vi "CRYCursor move in Cursor Table.vi"(8 "NewVal":string[][](array[string]), 9 "OldVal":string[][](array[string]), 10 "Cursor Coords":T1, 11 "pGraph VI":refnum<vi>) -> (3 "NewVal Out":string[][](array[string]))   [LabVIEW 2013]
uses:
  <vilib>/Utility/miscctls.llb/LVPoint32TypeDef.ctl
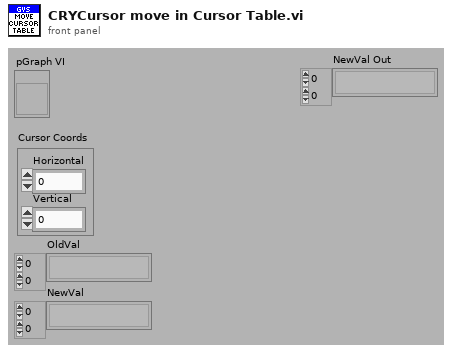
[diagram p1: front panel]
types:
  T1 = typedef "LVPoint32TypeDef.ctl" = cluster{"Horizontal":i32, "Vertical":i32}
  T2 = typedef "LVRowAndColumnTypeDef.ctl" = cluster{"Row":i32, "Column":i32}
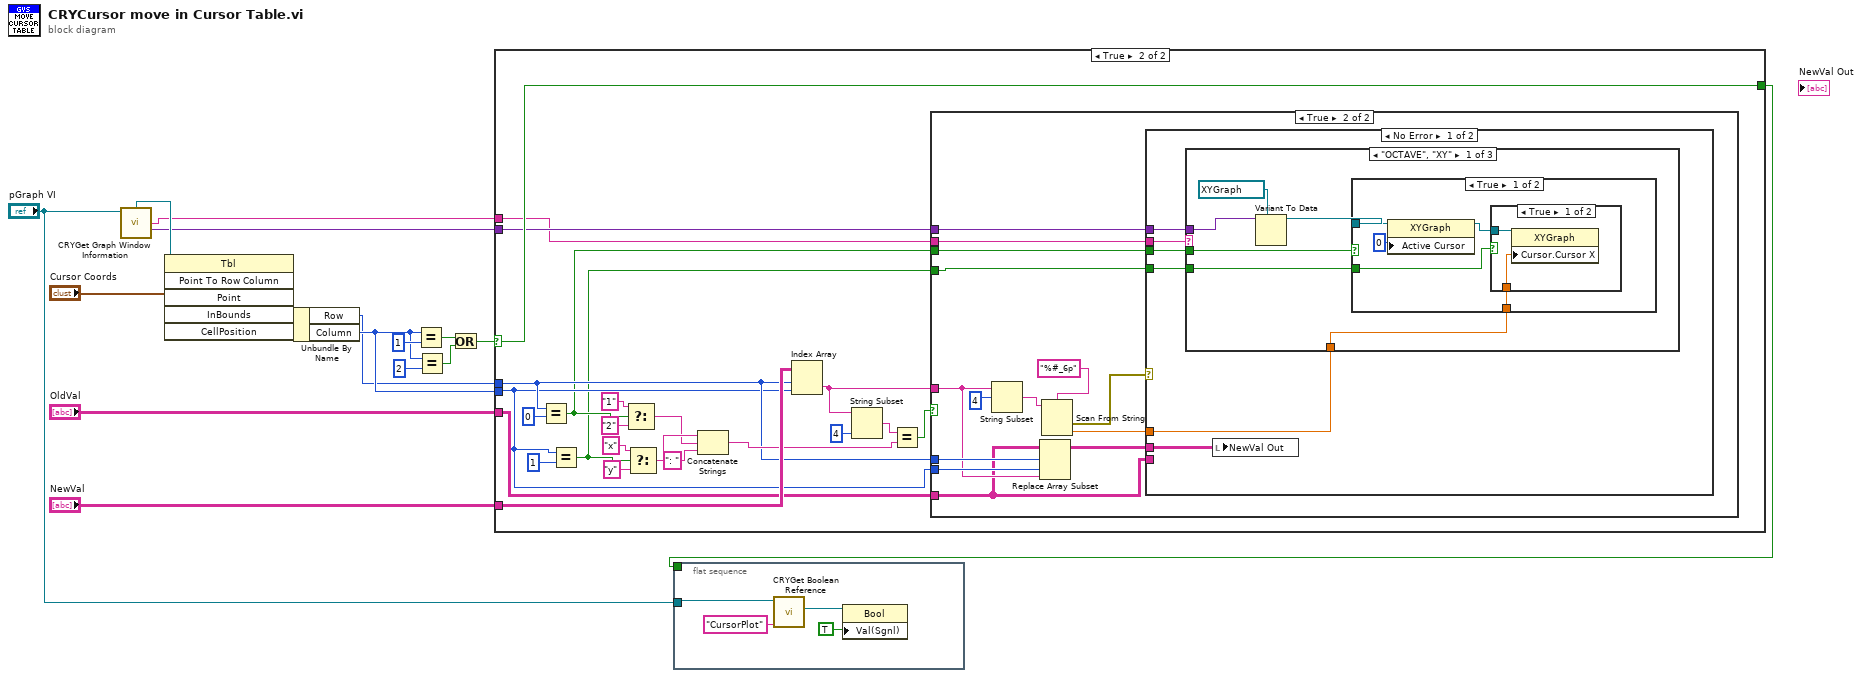
[diagram p0: block diagram]
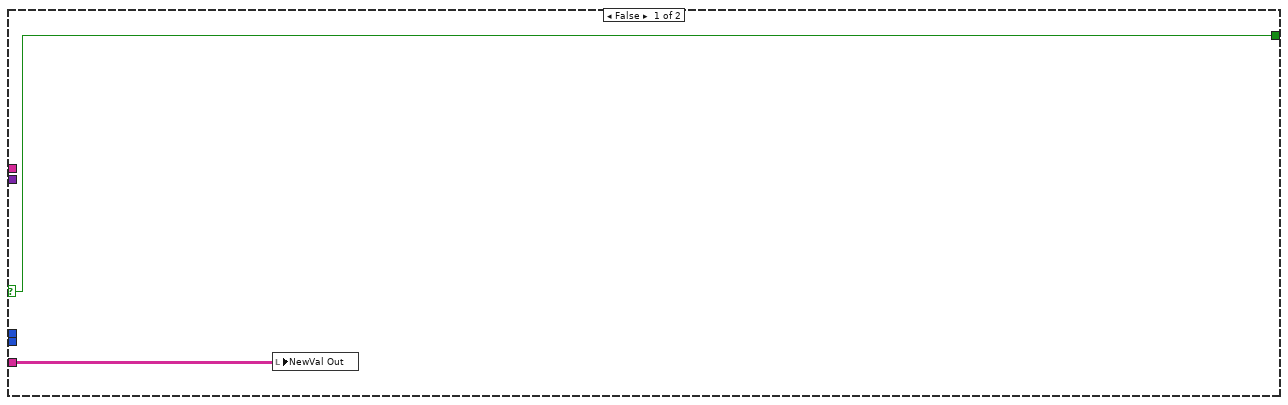
[diagram p2: hidden frame]
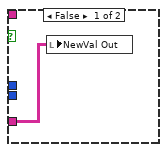
[diagram p3: hidden frame]
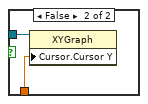
[diagram p4: hidden frame]
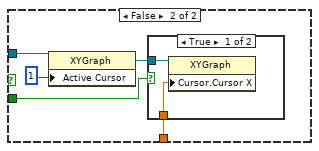
[diagram p5: hidden frame]
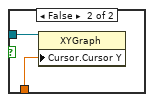
[diagram p6: hidden frame]
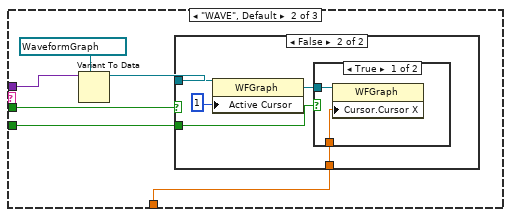
[diagram p7: hidden frame]
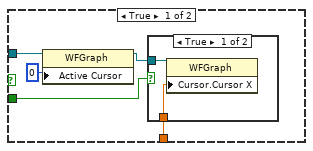
[diagram p8: hidden frame]
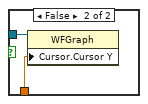
[diagram p9: hidden frame]
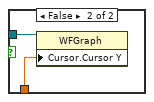
[diagram p10: hidden frame]
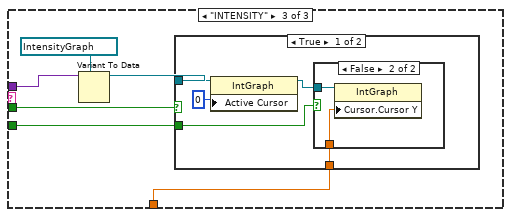
[diagram p11: hidden frame]
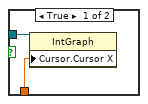
[diagram p12: hidden frame]
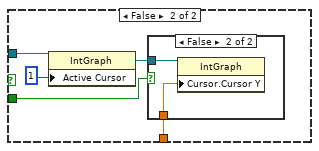
[diagram p13: hidden frame]
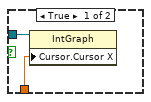
[diagram p14: hidden frame]
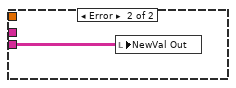
[diagram p15: hidden frame]
diagram:
  n1 = call "CRYGet Graph Window Information.vi"("pGraph VI In"="pGraph VI") -> ("Cursor Ref Out"=w5:refnum<vi>, "Graph Type Out"=w1:string, "Graph Control Ref Out"=w4:variant)  [unwired: 4 in, 8 out]
  n2 = invoke class="Tbl" method="Point To Row Column"(reference=w5, "Point"="Cursor Coords") -> ("CellPosition"=w11:T2)  [unwired: 4 in, 5 out]
  n3 = Unbundle By Name(w11) -> ("Row"=w12:i32, "Column"=w13:i32)
  n4 = Equal?(x=w13, y=1) -> (x = y?=w10:bool)
  n5 = Equal?(x=w13, y=2) -> (x = y?=w9:bool)
  n6 = Or(x=w10, y=w9) -> (x .or. y?=w16:bool)
  n7 = case shown="True" w16 {
    selector: w16 -> [w17 w24]
    tunnel: "NewVal" -> [_ w41]
    tunnel: w12 -> [_ w27]
    tunnel: w13 -> [_ w26]
    tunnel: "OldVal" -> [w18 w25]
    tunnel: [w17 w24] -> w2
    tunnel: w4 -> [_ w20]
    tunnel: w1 -> [_ w19]
    frame False {
      n8 = local write "NewVal Out"(w18) -> ()
    }
    frame True {
      n9 = Equal?(x=w27, y=0) -> (x = y?=w22:bool)
      n10 = Equal?(x=w26, y=1) -> (x = y?=w21:bool)
      n11 = Select(t="1", s=w22, f="2") -> (s? t:f=w33:string)
      n12 = Select(t="x", s=w21, f="y") -> (s? t:f=w34:string)
      n13 = Concatenate Strings(w34, w33, ": " ("string")) -> (w29:string)
      n14 = Index Array(array=w41, index (row)=w27, index (col)=w26) -> (element=w31:string)
      n15 = String Subset(string=w31, length (rest)=4 ("length (rest)")) -> (substring=w23:string)  [unwired: 1 in]
      n16 = Equal?(x=w23, y=w29) -> (x = y?=w28:bool)
      n17 = case shown="True" w28 {
        tunnel: w31 -> [_ w53]
        tunnel: w27 -> [_ w55]
        tunnel: w26 -> [_ w54]
        tunnel: w25 -> [w42 w43]
        tunnel: w22 -> [_ w49]
        tunnel: w21 -> [_ w48]
        tunnel: w19 -> [_ w46]
        tunnel: w20 -> [_ w45]
        frame False {
          n18 = local write "NewVal Out"(w42) -> ()
        }
        frame True {
          n19 = String Subset(string=w53, offset (0)=4) -> (substring=w51:string)  [unwired: 1 in]
          n20 = Replace Array Subset(array=w43, new element=w53, index (row)=w55, index (col)=w54) -> (w56:string[][])
          n21 = Scan From String(format string="%#_6p", input string=w51) -> (error out=w44:errorcluster, output 1=w47:dbl)  [unwired: 3 in, 2 out]
          n22 = case shown="No Error" w44 {
            tunnel: w56 -> [w62 _]
            tunnel: w49 -> [w61 _]
            tunnel: w48 -> [w60 _]
            tunnel: w47 -> [w59 _]
            tunnel: w46 -> [w58 _]
            tunnel: w45 -> [w57 _]
            tunnel: w43 -> [_ w135]
            frame No Error {
              n23 = case shown="\"OCTAVE\", \"XY\"" w58 {
                tunnel: w61 -> [w68 w92 w116]
                tunnel: w60 -> [w67 w91 w115]
                tunnel: w59 -> [w66 w90 w114]
                tunnel: w57 -> [w64 w88 w112]
                frame "OCTAVE", "XY" {
                  n24 = Variant To Data(type=refnum<vi> refnum ("GMListbox"), Variant=w64) -> (data=w63:refnum<vi>)  [unwired: 1 in, 1 out]
                  n25 = case shown="True" w68 {
                    tunnel: w67 -> [w71 w80]
                    tunnel: w66 -> [w73 w82]
                    tunnel: w63 -> [w70 w79]
                    frame True {
                      n26 = property on="Property Node" class="XYGraph"(reference=w70, "Active Cursor"=u32 0) -> (reference out=w69:refnum<vi>)  [unwired: 1 in, 1 out]
                      n27 = case shown="True" w71 {
                        tunnel: w73 -> [w75 w77]
                        tunnel: w69 -> [w74 w76]
                        frame True {
                          n28 = property on="Property Node" class="XYGraph"(reference=w74, "Cursor.Cursor X"=w75) -> ()  [unwired: 1 in, 2 out]
                        }
                        frame False {
                          n29 = property on="Property Node" class="XYGraph"(reference=w76, "Cursor.Cursor Y"=w77) -> ()  [unwired: 1 in, 2 out]
                        }
                      }
                    }
                    frame False {
                      n30 = property on="Property Node" class="XYGraph"(reference=w79, "Active Cursor"=u32 1) -> (reference out=w78:refnum<vi>)  [unwired: 1 in, 1 out]
                      n31 = case shown="True" w80 {
                        tunnel: w82 -> [w84 w86]
                        tunnel: w78 -> [w83 w85]
                        frame True {
                          n32 = property on="Property Node" class="XYGraph"(reference=w83, "Cursor.Cursor X"=w84) -> ()  [unwired: 1 in, 2 out]
                        }
                        frame False {
                          n33 = property on="Property Node" class="XYGraph"(reference=w85, "Cursor.Cursor Y"=w86) -> ()  [unwired: 1 in, 2 out]
                        }
                      }
                    }
                  }
                }
                frame "WAVE", Default {
                  n34 = Variant To Data(type=refnum<vi> refnum ("GMListbox"), Variant=w88) -> (data=w87:refnum<vi>)  [unwired: 1 in, 1 out]
                  n35 = case shown="False" w92 {
                    tunnel: w91 -> [w95 w104]
                    tunnel: w90 -> [w97 w106]
                    tunnel: w87 -> [w94 w103]
                    frame True {
                      n36 = property on="Property Node" class="WFGraph"(reference=w94, "Active Cursor"=u32 0) -> (reference out=w93:refnum<vi>)  [unwired: 1 in, 1 out]
                      n37 = case shown="True" w95 {
                        tunnel: w97 -> [w99 w101]
                        tunnel: w93 -> [w98 w100]
                        frame True {
                          n38 = property on="Property Node" class="WFGraph"(reference=w98, "Cursor.Cursor X"=w99) -> ()  [unwired: 1 in, 2 out]
                        }
                        frame False {
                          n39 = property on="Property Node" class="WFGraph"(reference=w100, "Cursor.Cursor Y"=w101) -> ()  [unwired: 1 in, 2 out]
                        }
                      }
                    }
                    frame False {
                      n40 = property on="Property Node" class="WFGraph"(reference=w103, "Active Cursor"=u32 1) -> (reference out=w102:refnum<vi>)  [unwired: 1 in, 1 out]
                      n41 = case shown="True" w104 {
                        tunnel: w106 -> [w108 w110]
                        tunnel: w102 -> [w107 w109]
                        frame True {
                          n42 = property on="Property Node" class="WFGraph"(reference=w107, "Cursor.Cursor X"=w108) -> ()  [unwired: 1 in, 2 out]
                        }
                        frame False {
                          n43 = property on="Property Node" class="WFGraph"(reference=w109, "Cursor.Cursor Y"=w110) -> ()  [unwired: 1 in, 2 out]
                        }
                      }
                    }
                  }
                }
                frame "INTENSITY" {
                  n44 = Variant To Data(type=refnum<vi> refnum ("GMListbox"), Variant=w112) -> (data=w111:refnum<vi>)  [unwired: 1 in, 1 out]
                  n45 = case shown="True" w116 {
                    tunnel: w115 -> [w119 w128]
                    tunnel: w114 -> [w121 w130]
                    tunnel: w111 -> [w118 w127]
                    frame True {
                      n46 = property on="Property Node" class="IntGraph"(reference=w118, "Active Cursor"=u32 0) -> (reference out=w117:refnum<vi>)  [unwired: 1 in, 1 out]
                      n47 = case shown="False" w119 {
                        tunnel: w121 -> [w123 w125]
                        tunnel: w117 -> [w122 w124]
                        frame True {
                          n48 = property on="Property Node" class="IntGraph"(reference=w122, "Cursor.Cursor X"=w123) -> ()  [unwired: 1 in, 2 out]
                        }
                        frame False {
                          n49 = property on="Property Node" class="IntGraph"(reference=w124, "Cursor.Cursor Y"=w125) -> ()  [unwired: 1 in, 2 out]
                        }
                      }
                    }
                    frame False {
                      n50 = property on="Property Node" class="IntGraph"(reference=w127, "Active Cursor"=u32 1) -> (reference out=w126:refnum<vi>)  [unwired: 1 in, 1 out]
                      n51 = case shown="False" w128 {
                        tunnel: w130 -> [w132 w134]
                        tunnel: w126 -> [w131 w133]
                        frame True {
                          n52 = property on="Property Node" class="IntGraph"(reference=w131, "Cursor.Cursor X"=w132) -> ()  [unwired: 1 in, 2 out]
                        }
                        frame False {
                          n53 = property on="Property Node" class="IntGraph"(reference=w133, "Cursor.Cursor Y"=w134) -> ()  [unwired: 1 in, 2 out]
                        }
                      }
                    }
                  }
                }
              }
              n54 = local write "NewVal Out"(w62) -> ()
            }
            frame Error {
              n55 = local write "NewVal Out"(w135) -> ()
            }
          }
        }
      }
    }
  }
  n56 = flat-sequence {
    tunnel: "pGraph VI" -> [w139]
    tunnel: w2 -> [_]
    frame #0 {
      n57 = call "CRYGet Boolean Reference.vi"("Label Name"="CursorPlot", "VI Refnum"=w139) -> ("Boolean Ref"=w137:refnum<vi>)  [unwired: 7 in, 2 out]
      n58 = property class="Bool"(reference=w137, "Val(Sgnl)"=TRUE ("Value (Signaling)")) -> ()  [unwired: 1 in, 2 out]
    }
  }
